vi "StandardEngineUI.vi"() -> ()   [LabVIEW 2013, in "Standard Engine Editor Node.lvclass"]
doc: "This VI is a template of the minimun components for a node UI.\nIt shows how to use the queue and the user event."
uses:
  Standard Engine Editor Node.lvclass
  <vilib>/NI/Configuration Framework/Node/NodeRef.ctl
  <vilib>/NI/Configuration Framework/Node/NISE_CEF_Node.lvclass
  <vilib>/NI/AMC/Message Queue.ctl
  <vilib>/NI/AMC/Message.ctl
  <vilib>/NI/Tools/Keyed Array/KeyedArray.ctl
  <vilib>/NI/Configuration Framework/Node/UserEventRef.ctl
  <vilib>/NI/Configuration Framework/Controls/EventCluster.ctl
  Execution Engine/Configuration/Supported Timing Sources.ctl
  Processor Assignment Mode.ctl
  Execution Engine/Configuration/Module Decimation.ctl
  Execution Engine/Configuration/timing reporting tags.ctl
  Execution Engine/Configuration/Error Actions By Category.ctl
  <vilib>/NI/Tag Bus Module Framework/runtime/error classification.ctl
  Execution Engine/Configuration/Error Actions.ctl
  <vilib>/NI/Tag Bus Data Framework/Configuration Editor/Classes/Engine Parent/Engine Parent Editor Node.lvclass
  Standard Engine Editor Node.lvclass/Standard Engine Editor Node.ctl
  Execution Engine/Configuration/Standard Engine Configuration.lvclass/Standard Engine Configuration.ctl
  Execution Engine/Configuration/Module Error Configuration.ctl
  Execution Engine/Configuration/Write Timing Source Type.vi
  Execution Engine/Configuration/Write Master Timing Module.vi
  Execution Engine/Configuration/Write Processor.vi
  Execution Engine/Configuration/Read Processor.vi
  Execution Engine/Configuration/Read Timing Source Type.vi
  <vilib>/NI/Tag Bus Data Framework/Configuration Editor/Classes/Engine Parent/Read Name.vi
  <vilib>/NI/AMC/Create Single Message.vi
  <vilib>/NI/AMC/Update Message Routing Info.vi
  <vilib>/NI/Configuration Framework/serializable configuration/get alias.vi
  Execution Engine/Configuration/Write Timing Source dt.vi
  Execution Engine/Configuration/Find Module Specific Config.vi
  <vilib>/Utility/error.llb/Error Cluster From Error Code.vi
  <vilib>/NI/Configuration Framework/error generator.vi
  <vilib>/NI/AMC/Send Message.vi
  Execution Engine/Configuration/Read Timing Source dt.vi
  <vilib>/NI/AMC/AMC.lvlib
  Execution Engine/Configuration/Standard Engine Configuration.lvclass
  <vilib>/NI/Tag Bus Module Framework/runtime/TBM module execution interface.lvclass
  <vilib>/NI/Configuration Framework/NISE_CEF_TreeControl.lvlib
  <vilib>/NI/Configuration Framework/serializable configuration/NISE_CEF_serializable configuration.lvclass
  <vilib>/NI/Tools/Keyed Array/Tools_KeyedArray.lvlib
panel:
  in  "Tab Control":T1(tab)
  in  "Enable Timing Report":bool
  in  "Module Timing Source":i32(listbox)
  in  "Engine Name":string
  in  "Timing Source dt":u32=5000
  in  "Timing Source Type":T2=enum."1 kHz Clock"
  in  "Procesor Assignment":i32 min=0
  in  "Mode":T3
  in  "Warning Message":string="This timing source is not deterministic."
  out "timing reporting":T4={"late index (bool)"="_stdeng_late", "late count index (U32)"="_stdeng_latecount", "current dt ns(U64)"="_stdeng_iteratedt"}
  in  "Report Errors?":bool
  out "error tag":string
  in  "Module to Configure":i32(listbox)
  in  "Module Decimation":T5={"Decimation"=1, "Offset"=0} {"Decimation" min=1}
  in  "Sort Order":i32
  in  "Async?":bool
  in  "Error Handling":T6[](array[typedef])
  in  "user event":T9
  in  "main queue":T10
  in  "node ref":T11
  # "Processor Assignment"
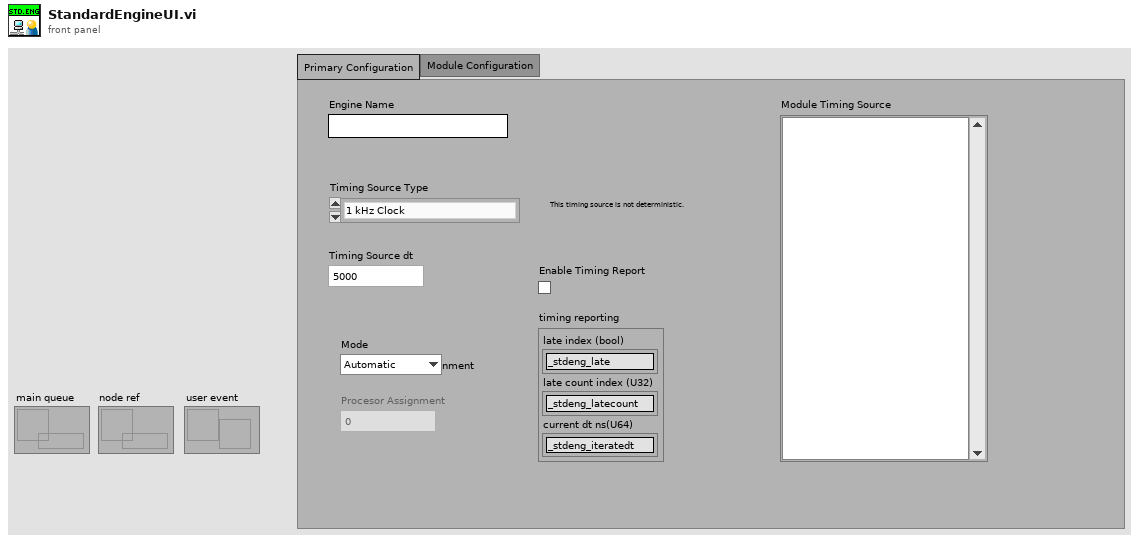
[diagram p1: front panel]
types:
  T1 = enum32{"Primary Configuration", "Module Configuration"}
  T2 = typedef "Standard Engine Configuration.lvclass/Supported Timing Sources.ctl" = enum16{"Use Module Timing Source", "1 kHz Clock", "1 MHz Clock", "Synchronize to Scan Engine"}
  T3 = typedef "Standard Engine Editor Node.lvclass/Processor Assignment Mode.ctl" = enum16{"Automatic", "Manual"}
  T4 = typedef "Standard Engine Configuration.lvclass/timing reporting tags.ctl" = cluster{"late index (bool)":string, "late count index (U32)":string, "current dt ns(U64)":string}
  T5 = typedef "Standard Engine Configuration.lvclass/Module Decimation.ctl" = cluster{"Decimation":u16, "Offset":u16}
  T6 = typedef "Standard Engine Configuration.lvclass/Error Actions By Category.ctl" = cluster{"error classification":T7, "Error Actions":T8[]}
  T7 = typedef "TBM module execution interface.lvclass/error classification.ctl" = enum16{"unknown", "none", "trivial", "recoverable", "critical"}
  T8 = typedef "Standard Engine Configuration.lvclass/Error Actions.ctl" = enum16{"Clear", "Notify", "Stop Component", "Stop Engine", "Safe State", "Attempt Recovery"}
  T9 = typedef "NISE_CEF_Node.lvclass/UserEventRef.ctl" = refnum<user-event>
  T10 = typedef "AMC.lvlib/Message Queue.ctl" = refnum<queue>
  T11 = typedef "NISE_CEF_Node.lvclass/NodeRef.ctl" = refnum<data-value>
  T12 = typedef "NISE_CEF_TreeControl.lvlib/EventCluster.ctl" = cluster{"command":string, "data":string}
  T13 = typedef "Standard Engine Configuration.lvclass/Module Error Configuration.ctl" = cluster{"Module Error Configuration":T6[]}
  T14 = enum8{"Enabled", "Disabled", "Disabled and Grayed Out"}
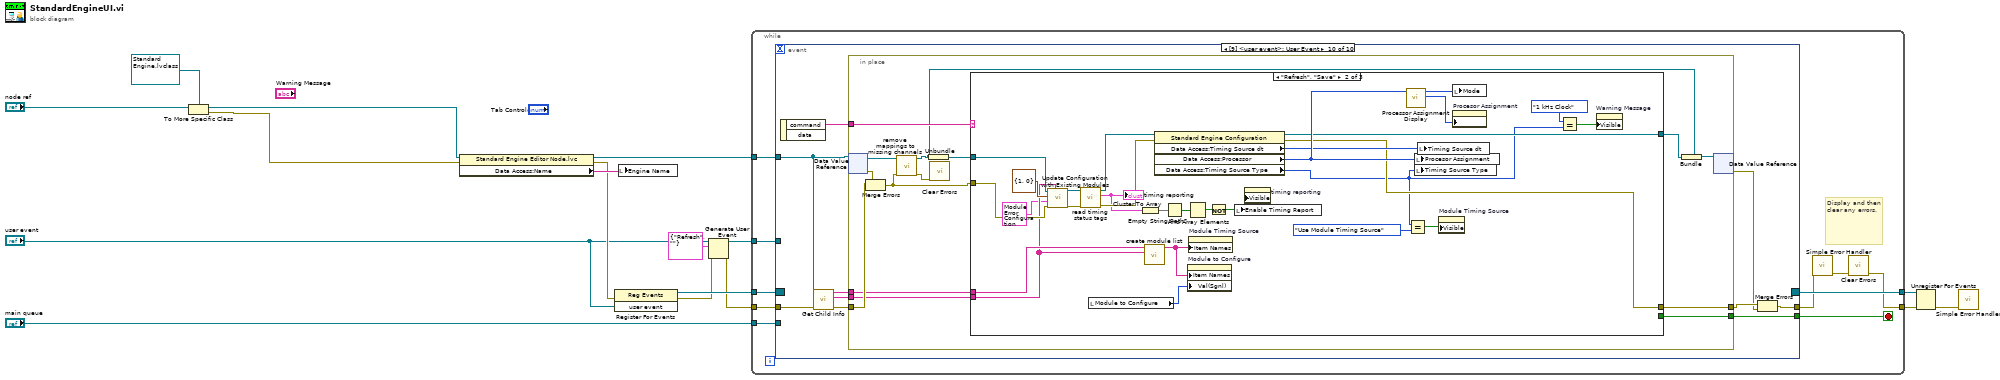
[diagram p0: block diagram]
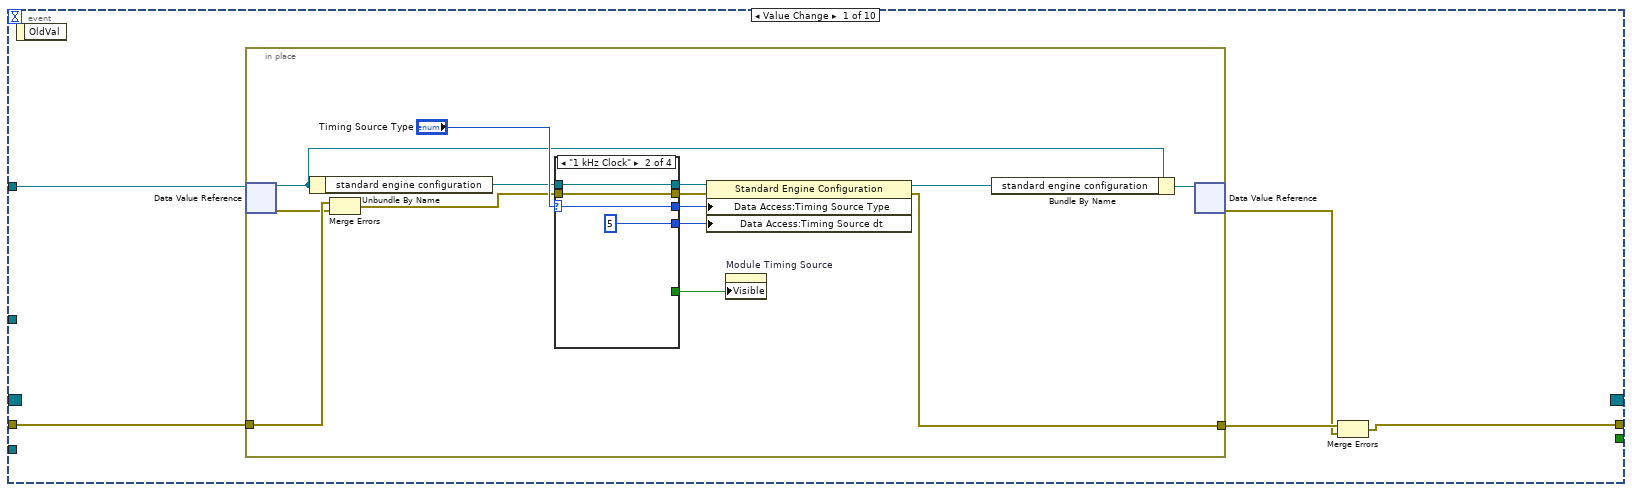
[diagram p2: hidden frame]
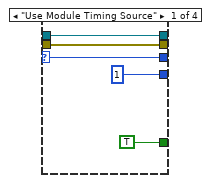
[diagram p3: hidden frame]
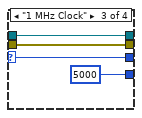
[diagram p4: hidden frame]
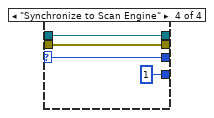
[diagram p5: hidden frame]
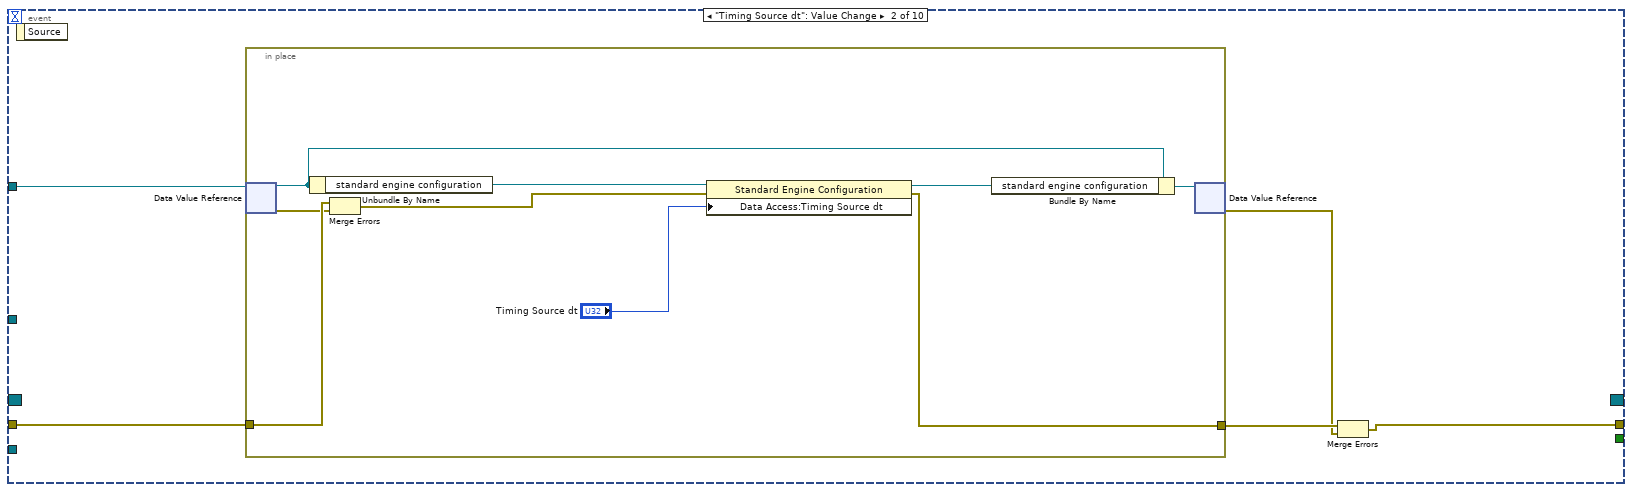
[diagram p6: hidden frame]
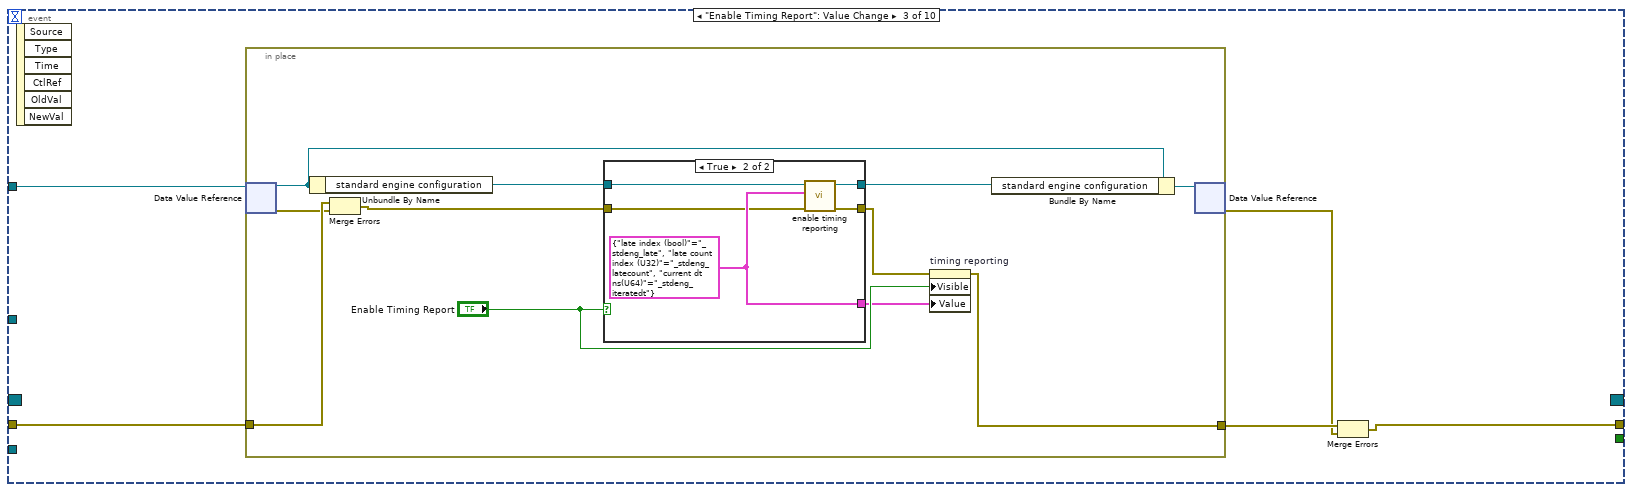
[diagram p7: hidden frame]
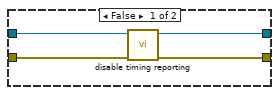
[diagram p8: hidden frame]
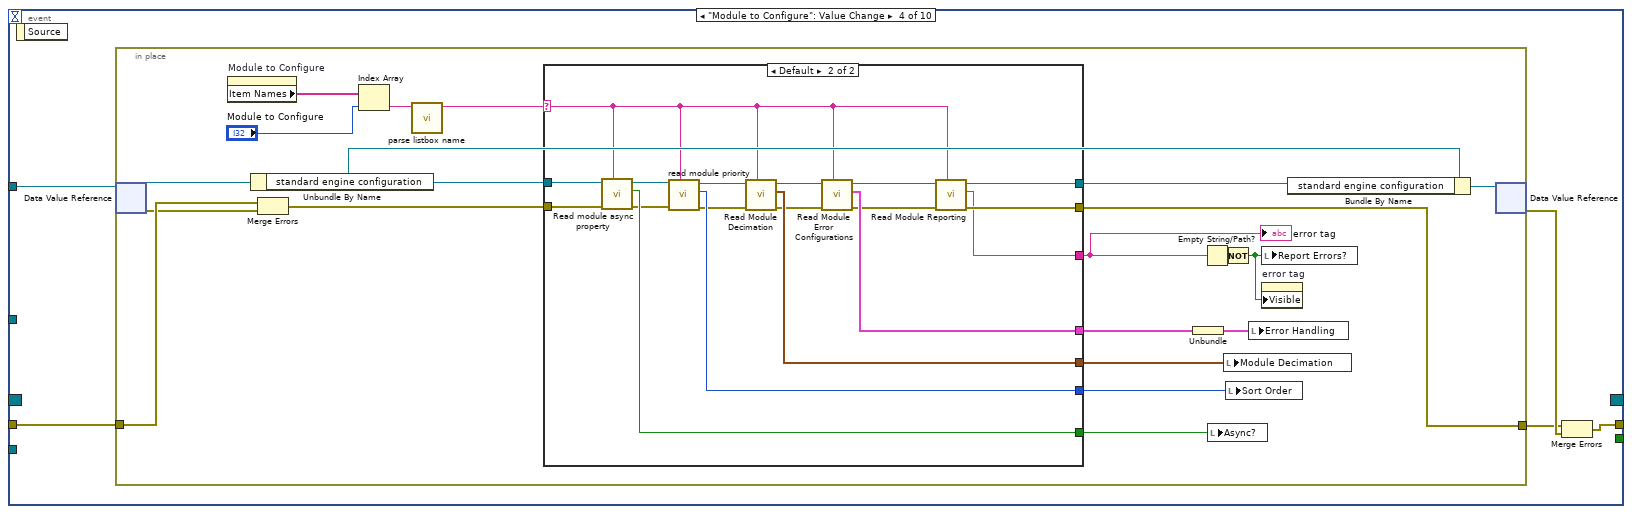
[diagram p9: hidden frame]
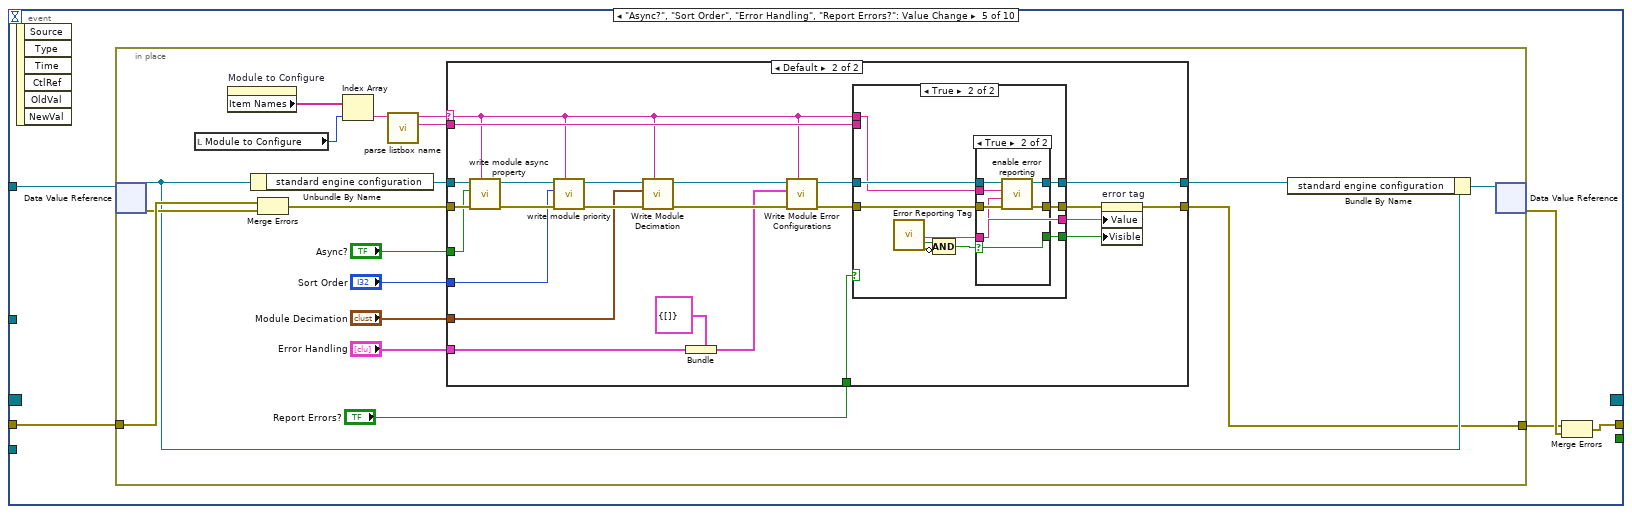
[diagram p11: hidden frame]
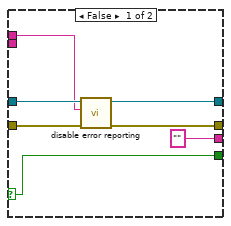
[diagram p13: hidden frame]
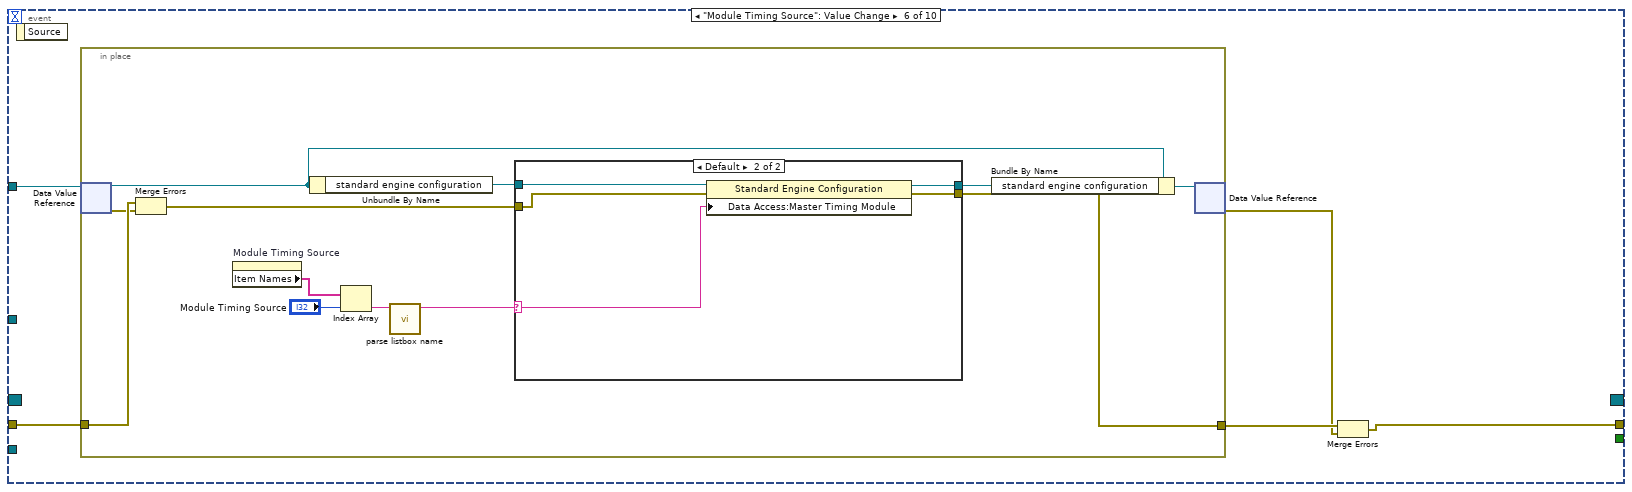
[diagram p15: hidden frame]
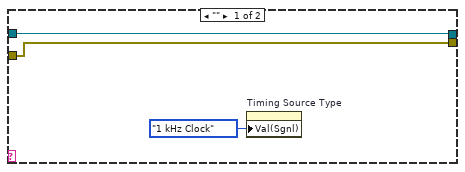
[diagram p16: hidden frame]
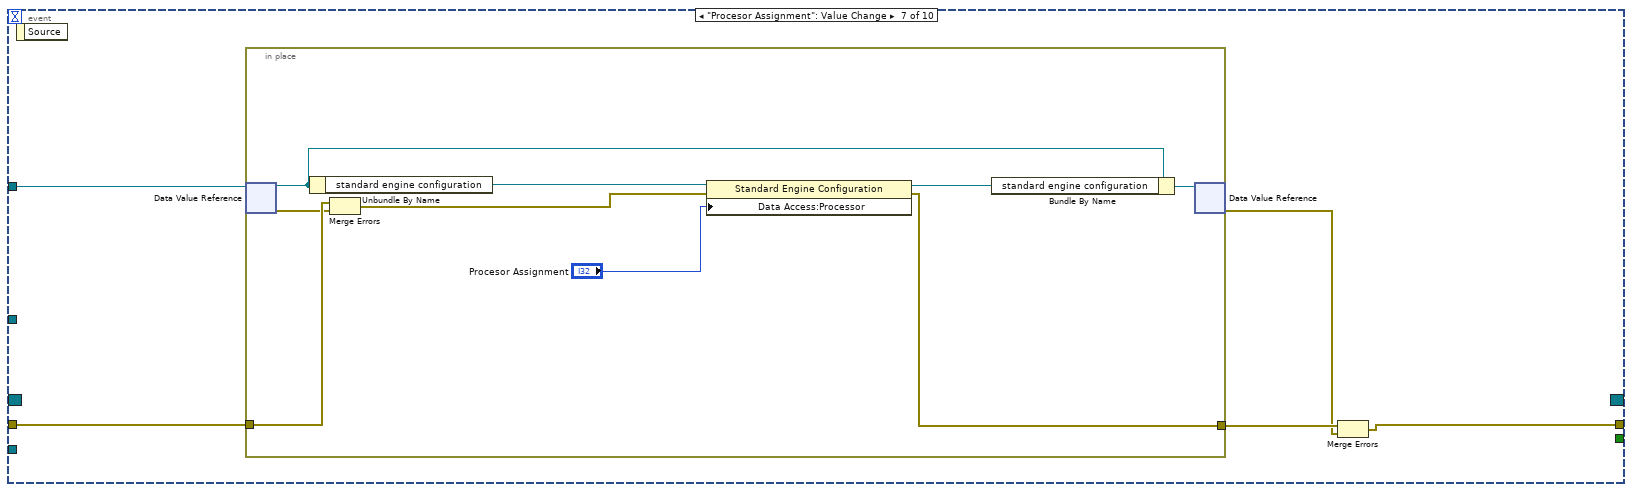
[diagram p17: hidden frame]
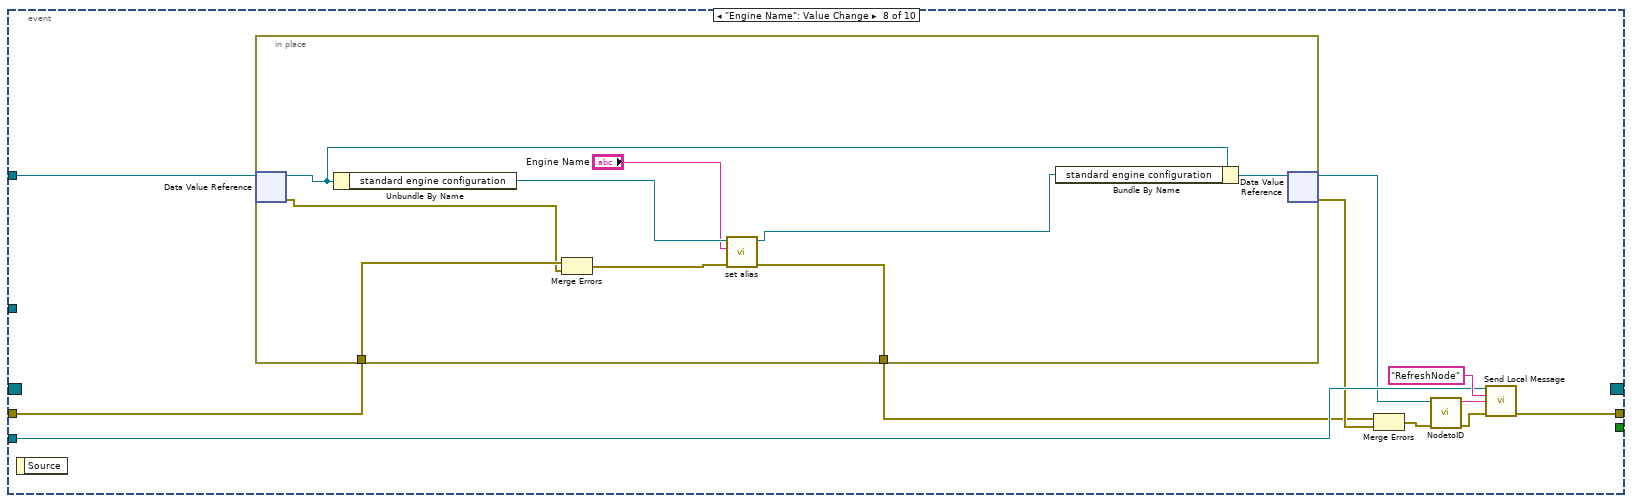
[diagram p18: hidden frame]
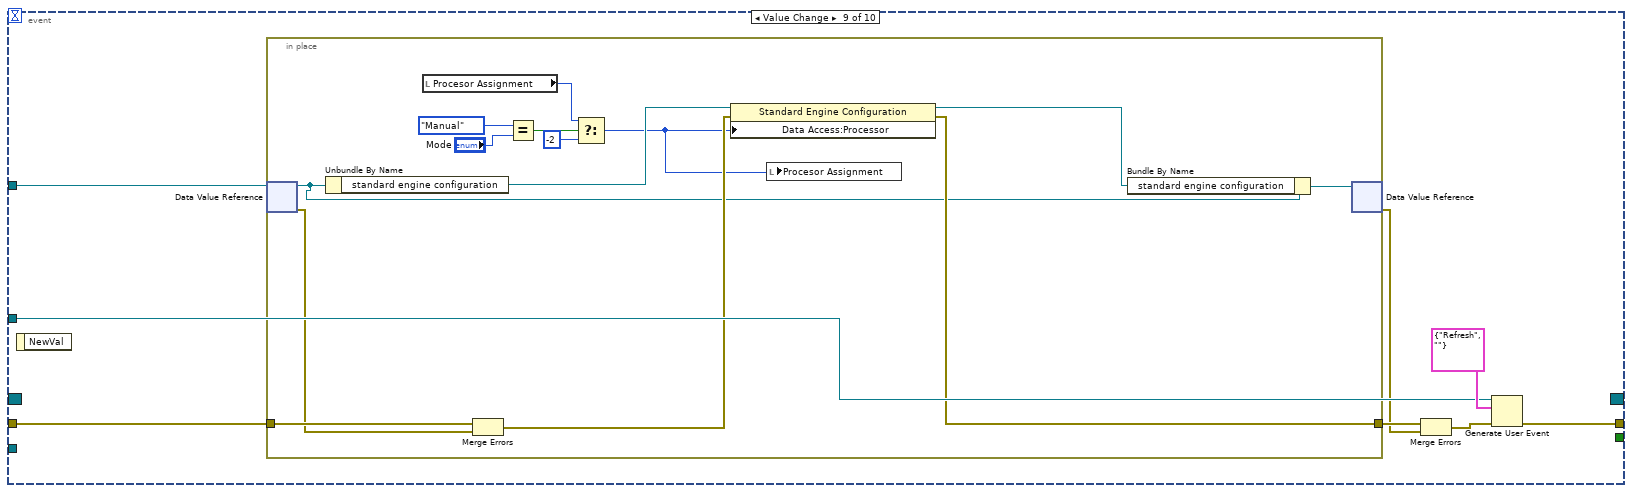
[diagram p19: hidden frame]
diagram:
  n1 = To More Specific Class(target class=refnum<data-value> refnum ("data value reference"), reference="node ref") -> (specific class reference=w12:refnum<data-value>, error out=w11:errorcluster)  [unwired: 1 in]
  n2 = property class="Standard Engine Editor Node.lvc"(reference=w12, error in=w11) -> (reference out=w8:refnum<data-value>, error out=w7:errorcluster, "Data Access:Name"=w13:string)
  n3 = register-events(error in=w7, "user event") -> (reference out=w16:refnum<event-registration>, error out=w6:errorcluster)  [unwired: 1 in]
  n4 = local write "Engine Name"(w13) -> ()
  n5 = Generate User Event(user event="user event", event data cluster=T12 {"command"="Refresh", "data"=""} ("event data"), error in=w6) -> (user event out=w3:T9, error out=w5:errorcluster)  [unwired: 1 in]
  n6 = while {
    tunnel: "main queue" -> [w27]
    tunnel: w16 -> [w26]
    tunnel: [w25] -> w15
    tunnel: [w19] -> w14
    tunnel: w5 -> [w23]
    tunnel: w8 -> [w22]
    tunnel: w3 -> [w18]
    stop <- w24 stop-if-true
    # "Display and then clear any errors."
    n7 = event shown="[9] <user event>: User Event" {
      selector: w26 -> [_ _ _ _ _ _ _ _ _ _]
      dyn-events: [_ _ _ _ _ _ _ _ _ _] -> w25
      timeout: _ -> [_ _ _ _ _ _ _ _ _ _]
      tunnel: w27 -> [_ _ _ _ _ _ _ w272 _ _]
      tunnel: [_ _ _ _ _ _ _ _ _ w314] -> w24
      tunnel: [w29 w65 w79 w105 w150 w225 w250 w270 w287 w306] -> w21
      tunnel: w23 -> [w32 w68 w82 w107 w152 w228 w253 w268 w286 w309]
      tunnel: w22 -> [w30 w66 w80 w106 w151 w226 w251 w267 w284 w307]
      tunnel: w18 -> [_ _ _ _ _ _ _ _ w289 _]
      event Value Change {
        n8 = event-data() -> ()  [unwired: 1 in, 1 out]
        n9 = in-place {
          in-place-border: w32 -> [w45]
          in-place-border: [w41] -> w31
          n10 = in-place-dvr #1(w30) -> (w36:refnum<class "Standard Engine Editor Node.lvclass">, w38:errorcluster)
          n11 = Unbundle By Name(w36) -> ("standard engine configuration"=w37:refnum<class "Standard Engine Configuration.lvclass">)
          n12 = Merge Errors(w45, w38) -> (w39:errorcluster)
          n13 = case shown="\"1 kHz Clock\"" "Timing Source Type" {
            selector: "Timing Source Type" -> [w51 w55 w57 w61]
            tunnel: w37 -> [w50 w54 w59 w63]
            tunnel: [w50 w54 w59 w63] -> w46
            tunnel: w39 -> [w49 w53 w58 w62]
            tunnel: [w49 w53 w58 w62] -> w44
            tunnel: [w51 w55 w57 w61] -> w40
            tunnel: [u32 1 ("Timing Source dt") u32 5 ("Timing Source dt") u32 5000 ("Timing Source dt") u32 1 ("Timing Source dt")] -> w42
            tunnel: [TRUE _ _ _] -> w33
            frame "Use Module Timing Source" {
            }
            frame "1 kHz Clock" {
            }
            frame "1 MHz Clock" {
            }
            frame "Synchronize to Scan Engine" {
            }
          }
          n14 = property class="Standard Engine Configuration"(reference=w46, error in=w44, "Data Access:Timing Source Type"=w40, "Data Access:Timing Source dt"=w42) -> (reference out=w34:refnum<class "Standard Engine Configuration.lvclass">, error out=w41:errorcluster)
          n15 = property on="Module Timing Source" class="LstBox (strict)"("Visible"=w33) -> ()  [unwired: 2 in, 2 out]
          n16 = Bundle By Name(cluster=w36, "standard engine configuration"=w34) -> (w35:refnum<class "Standard Engine Editor Node.lvclass">)
          n17 = in-place-dvr #1(w35) -> (w28:errorcluster)  [unwired: 1 out]
        }
        n18 = Merge Errors(w31, w28) -> (w29:errorcluster)
      }
      event "Timing Source dt": Value Change {
        n19 = event-data() -> ()  [unwired: 1 in, 1 out]
        n20 = in-place {
          in-place-border: w68 -> [w77]
          in-place-border: [w76] -> w67
          n21 = in-place-dvr #2(w66) -> (w72:refnum<class "Standard Engine Editor Node.lvclass">, w74:errorcluster)
          n22 = Unbundle By Name(w72) -> ("standard engine configuration"=w73:refnum<class "Standard Engine Configuration.lvclass">)
          n23 = Merge Errors(w77, w74) -> (w75:errorcluster)
          n24 = property class="Standard Engine Configuration"(reference=w73, error in=w75, "Data Access:Timing Source dt"="Timing Source dt") -> (reference out=w70:refnum<class "Standard Engine Configuration.lvclass">, error out=w76:errorcluster)
          n25 = Bundle By Name(cluster=w72, "standard engine configuration"=w70) -> (w71:refnum<class "Standard Engine Editor Node.lvclass">)
          n26 = in-place-dvr #2(w71) -> (w64:errorcluster)  [unwired: 1 out]
        }
        n27 = Merge Errors(w67, w64) -> (w65:errorcluster)
      }
      event "Enable Timing Report": Value Change {
        n28 = event-data() -> ()  [unwired: 1 in, 6 out]
        n29 = in-place {
          in-place-border: w82 -> [w93]
          in-place-border: [w89] -> w81
          n30 = in-place-dvr #3(w80) -> (w91:refnum<class "Standard Engine Editor Node.lvclass">, w92:errorcluster)
          n31 = Unbundle By Name(w91) -> ("standard engine configuration"=w87:refnum<class "Standard Engine Configuration.lvclass">)
          n32 = Merge Errors(w93, w92) -> (w84:errorcluster)
          n33 = case shown="True" "Enable Timing Report" {
            tunnel: w87 -> [w97 w102]
            tunnel: [w95 w101] -> w86
            tunnel: [_ w100] -> w85
            tunnel: w84 -> [w96 w99]
            tunnel: [w94 w98] -> w83
            frame False {
              n34 = call "disable timing reporting.vi"("error in"=w96, "Standard Engine Configuration in"=w97) -> ("error out"=w94:errorcluster, "Standard Engine Configuration out"=w95:refnum<class "Standard Engine Configuration.lvclass">)  [unwired: 8 in]
            }
            frame True {
              w100 = T4 {"late index (bool)"="_stdeng_late", "late count index (U32)"="_stdeng_latecount", "current dt ns(U64)"="_stdeng_iteratedt"} ("timing reporting")
              n35 = call "enable timing reporting.vi"("error in"=w99, "timing reporting"=w100, "Standard Engine Configuration in"=w102) -> ("error out"=w98:errorcluster, "Standard Engine Configuration out"=w101:refnum<class "Standard Engine Configuration.lvclass">)  [unwired: 7 in]
            }
          }
          n36 = property on="timing reporting" class="Clust (strict)"(error in=w83, "Visible"="Enable Timing Report", "Value"=w85) -> (error out=w89:errorcluster)  [unwired: 1 in, 1 out]
          n37 = Bundle By Name(cluster=w91, "standard engine configuration"=w86) -> (w90:refnum<class "Standard Engine Editor Node.lvclass">)
          n38 = in-place-dvr #3(w90) -> (w78:errorcluster)  [unwired: 1 out]
        }
        n39 = Merge Errors(w81, w78) -> (w79:errorcluster)
      }
      event "Module to Configure": Value Change {
        n40 = event-data() -> ()  [unwired: 1 in, 1 out]
        n41 = in-place {
          in-place-border: w107 -> [w127]
          in-place-border: [w112] -> w103
          n42 = in-place-dvr #4(w106) -> (w125:refnum<class "Standard Engine Editor Node.lvclass">, w126:errorcluster)
          n43 = property on="Module to Configure" class="LstBox (strict)"() -> ("Item Names"=w123:string[])  [unwired: 2 in, 2 out]
          n44 = Unbundle By Name(w125) -> ("standard engine configuration"=w120:refnum<class "Standard Engine Configuration.lvclass">)
          n45 = Merge Errors(w127, w126) -> (w119:errorcluster)
          n46 = Index Array(array=w123, index="Module to Configure") -> (element=w121:string)
          n47 = call "parse listbox name.vi"("formatted name"=w121) -> ("ID"=w108:string)  [unwired: 9 in, 1 out]
          n48 = case shown="Default" w108 {
            selector: w108 -> [_ w130]
            tunnel: w120 -> [w129 w147]
            tunnel: w119 -> [w128 w146]
            tunnel: [_ w145] -> w118
            tunnel: [_ w142] -> w117
            tunnel: [_ w139] -> w116
            tunnel: [_ w136] -> w115
            tunnel: [w128 w133] -> w112
            tunnel: [w129 w132] -> w111
            tunnel: [_ w131] -> w110
            frame "" {
            }
            frame Default {
              n49 = call "Read module async property.vi"("Module ID"=w130, "error in"=w146, "Standard Engine Repo Data in"=w147) -> ("error out"=w143:errorcluster, "async?"=w145:bool, "Standard Engine Repo Data out"=w144:refnum<class "Standard Engine Configuration.lvclass">)  [unwired: 6 in]
              n50 = call "read module priority.vi"("Module ID"=w130, "error in"=w143, "Standard Engine Repo Data in"=w144) -> ("error out"=w141:errorcluster, "execution order priority"=w142:i32, "Standard Engine Repo Data out"=w140:refnum<class "Standard Engine Configuration.lvclass">)  [unwired: 6 in]
              n51 = call "Read Module Decimation.vi"("Module ID"=w130, "error in"=w141, "Standard Engine Repo Data in"=w140) -> ("error out"=w137:errorcluster, "Module Decimation"=w139:T5, "Standard Engine Repo Data out"=w138:refnum<class "Standard Engine Configuration.lvclass">)  [unwired: 6 in]
              n52 = call "Read Module Error Configurations.vi"("Module ID"=w130, "error in"=w137, "Standard Engine Repo Data in"=w138) -> ("error out"=w134:errorcluster, "Module Error Configuration"=w136:T13, "Standard Engine Repo Data out"=w135:refnum<class "Standard Engine Configuration.lvclass">)  [unwired: 6 in]
              n53 = call "Read Module Reporting.vi"("Module ID"=w130, "error in"=w134, "Standard Engine Repo Data in"=w135) -> ("error out"=w133:errorcluster, "error tag"=w131:string, "Standard Engine Repo Data out"=w132:refnum<class "Standard Engine Configuration.lvclass">)  [unwired: 6 in]
            }
          }
          "error tag" <- w110
          n54 = Unbundle(w115) -> ("Module Error Configuration"=w114:T6[])
          n55 = Empty String/Path?(string/path=w110) -> (empty?=w113:bool)
          n56 = local write "Async?"(w118) -> ()
          n57 = Not(x=w113) -> (.not. x?=w109:bool)
          n58 = local write "Module Decimation"(w116) -> ()
          n59 = local write "Sort Order"(w117) -> ()
          n60 = local write "Error Handling"(w114) -> ()
          n61 = local write "Report Errors?"(w109) -> ()
          n62 = property on="error tag" class="Str"("Visible"=w109) -> ()  [unwired: 2 in, 2 out]
          n63 = Bundle By Name(cluster=w125, "standard engine configuration"=w111) -> (w124:refnum<class "Standard Engine Editor Node.lvclass">)
          n64 = in-place-dvr #4(w124) -> (w104:errorcluster)  [unwired: 1 out]
        }
        n65 = Merge Errors(w103, w104) -> (w105:errorcluster)
      }
      event "Async?", "Sort Order", "Error Handling", "Report Errors?": Value Change {
        n66 = event-data() -> ()  [unwired: 1 in, 6 out]
        n67 = in-place {
          in-place-border: w152 -> [w170]
          in-place-border: [w156] -> w148
          n68 = in-place-dvr #5(w151) -> (w168:refnum<class "Standard Engine Editor Node.lvclass">, w169:errorcluster)
          n69 = local read "Module to Configure"() -> (w159:i32)
          n70 = property on="Module to Configure" class="LstBox (strict)"() -> ("Item Names"=w166:string[])  [unwired: 2 in, 2 out]
          n71 = Unbundle By Name(w168) -> ("standard engine configuration"=w164:refnum<class "Standard Engine Configuration.lvclass">)
          n72 = Merge Errors(w170, w169) -> (w163:errorcluster)
          n73 = Index Array(array=w166, index=w159) -> (element=w165:string)
          n74 = call "parse listbox name.vi"("formatted name"=w165) -> ("display"=w154:string, "ID"=w153:string)  [unwired: 9 in]
          n75 = case shown="Default" w153 {
            selector: w153 -> [_ w174]
            tunnel: w164 -> [w172 w196]
            tunnel: w163 -> [w171 w195]
            tunnel: "Async?" -> [_ w190]
            tunnel: "Sort Order" -> [_ w189]
            tunnel: "Module Decimation" -> [_ w188]
            tunnel: [w172 w183] -> w158
            tunnel: "Error Handling" -> [_ w181]
            tunnel: [w171 w179] -> w156
            tunnel: "Report Errors?" -> [_ w177]
            tunnel: w154 -> [_ w175]
            frame "" {
            }
            frame Default {
              n76 = call "write module async property.vi"("Module ID"=w174, "error in"=w195, "async?"=w190, "Standard Engine Repo Data in"=w196) -> ("error out"=w193:errorcluster, "Standard Engine Repo Data out"=w194:refnum<class "Standard Engine Configuration.lvclass">)  [unwired: 6 in]
              n77 = call "write module priority.vi"("Module ID"=w174, "error in"=w193, "execution order priority"=w189, "Standard Engine Repo Data in"=w194) -> ("error out"=w191:errorcluster, "Standard Engine Repo Data out"=w192:refnum<class "Standard Engine Configuration.lvclass">)  [unwired: 6 in]
              n78 = call "Write Module Decimation.vi"("Module ID"=w174, "error in"=w191, "Module Decimation"=w188, "Standard Engine Repo Data in"=w192) -> ("error out"=w186:errorcluster, "Standard Engine Repo Data out"=w187:refnum<class "Standard Engine Configuration.lvclass">)  [unwired: 6 in]
              n79 = Bundle(cluster=T13 {"Module Error Configuration"=[]} ("Module Error Configuration"), "Module Error Configuration"=w181) -> (w180:T13)
              n80 = call "Write Module Error Configurations.vi"("Module ID"=w174, "error in"=w186, "Module Error Configuration"=w180, "Standard Engine Repo Data in"=w187) -> ("error out"=w184:errorcluster, "Standard Engine Repo Data out"=w185:refnum<class "Standard Engine Configuration.lvclass">)  [unwired: 6 in]
              n81 = case shown="True" w177 {
                selector: w177 -> [w197 _]
                tunnel: w185 -> [w203 w213]
                tunnel: w184 -> [w202 w212]
                tunnel: [w200 w211] -> w183
                tunnel: [w201 w210] -> w178
                tunnel: w174 -> [w199 w209]
                tunnel: ["" w208] -> w176
                tunnel: w175 -> [_ _]
                tunnel: [w197 w204] -> w173
                frame False {
                  n82 = call "disable error reporting.vi"("error in"=w202, "module ID"=w199, "Standard Engine Configuration in"=w203) -> ("error out"=w201:errorcluster, "Standard Engine Configuration out"=w200:refnum<class "Standard Engine Configuration.lvclass">)  [unwired: 7 in]
                }
                frame True {
                  n83 = call "Error Reporting Tag"() -> ("Tag Name"=w208:string, "OK"=w207:bool, "error out"=w206:errorcluster)  [unwired: 17 in]
                  n84 = Compound Arithmetic op=AND(w207, invert w206) -> (w205:bool)
                  n85 = case shown="True" w205 {
                    selector: w205 -> [w214 w217]
                    tunnel: w213 -> [w216 w223]
                    tunnel: w212 -> [w215 w222]
                    tunnel: [w216 w221] -> w211
                    tunnel: [w215 w220] -> w210
                    tunnel: w209 -> [_ w219]
                    tunnel: w208 -> [_ w218]
                    tunnel: [w214 w217] -> w204
                    frame False {
                    }
                    frame True {
                      n86 = call "enable error reporting.vi"("error in"=w222, "tag"=w218, "module ID"=w219, "Standard Engine Configuration in"=w223) -> ("error out"=w220:errorcluster, "Standard Engine Configuration out"=w221:refnum<class "Standard Engine Configuration.lvclass">)  [unwired: 6 in]
                    }
                  }
                }
              }
              n87 = property on="error tag" class="Str"(error in=w178, "Value"=w176, "Visible"=w173) -> (error out=w179:errorcluster)  [unwired: 1 in, 1 out]
            }
          }
          n88 = Bundle By Name(cluster=w168, "standard engine configuration"=w158) -> (w167:refnum<class "Standard Engine Editor Node.lvclass">)
          n89 = in-place-dvr #5(w167) -> (w149:errorcluster)  [unwired: 1 out]
        }
        n90 = Merge Errors(w148, w149) -> (w150:errorcluster)
      }
      event "Module Timing Source": Value Change {
        n91 = event-data() -> ()  [unwired: 1 in, 1 out]
        n92 = in-place {
          in-place-border: w228 -> [w240]
          in-place-border: [w239] -> w227
          n93 = in-place-dvr #6(w226) -> (w235:refnum<class "Standard Engine Editor Node.lvclass">, w237:errorcluster)
          n94 = Merge Errors(w240, w237) -> (w238:errorcluster)
          n95 = property on="Module Timing Source" class="LstBox (strict)"() -> ("Item Names"=w231:string[])  [unwired: 2 in, 2 out]
          n96 = Unbundle By Name(w235) -> ("standard engine configuration"=w236:refnum<class "Standard Engine Configuration.lvclass">)
          n97 = Index Array(array=w231, index="Module Timing Source") -> (element=w230:string)
          n98 = call "parse listbox name.vi"("formatted name"=w230) -> ("ID"=w229:string)  [unwired: 9 in, 1 out]
          n99 = case shown="Default" w229 {
            selector: w229 -> [_ w244]
            tunnel: [w243 w248] -> w239
            tunnel: w238 -> [w243 w247]
            tunnel: w236 -> [w242 w246]
            tunnel: [w242 w245] -> w233
            frame "" {
              n100 = property on="Timing Source Type" class="Enum (strict)"("Val(Sgnl)"=Supported_Timing_Sources."1 kHz Clock" ("Value (Signaling)")) -> ()  [unwired: 2 in, 2 out]
            }
            frame Default {
              n101 = property class="Standard Engine Configuration"(reference=w246, error in=w247, "Data Access:Master Timing Module"=w244) -> (reference out=w245:refnum<class "Standard Engine Configuration.lvclass">, error out=w248:errorcluster)
            }
          }
          n102 = Bundle By Name(cluster=w235, "standard engine configuration"=w233) -> (w234:refnum<class "Standard Engine Editor Node.lvclass">)
          n103 = in-place-dvr #6(w234) -> (w224:errorcluster)  [unwired: 1 out]
        }
        n104 = Merge Errors(w227, w224) -> (w225:errorcluster)
      }
      event "Procesor Assignment": Value Change {
        n105 = event-data() -> ()  [unwired: 1 in, 1 out]
        n106 = in-place {
          in-place-border: w253 -> [w262]
          in-place-border: [w261] -> w252
          n107 = in-place-dvr #7(w251) -> (w257:refnum<class "Standard Engine Editor Node.lvclass">, w259:errorcluster)
          n108 = Unbundle By Name(w257) -> ("standard engine configuration"=w258:refnum<class "Standard Engine Configuration.lvclass">)
          n109 = Merge Errors(w262, w259) -> (w260:errorcluster)
          n110 = property class="Standard Engine Configuration"(reference=w258, error in=w260, "Data Access:Processor"="Procesor Assignment") -> (reference out=w255:refnum<class "Standard Engine Configuration.lvclass">, error out=w261:errorcluster)
          n111 = Bundle By Name(cluster=w257, "standard engine configuration"=w255) -> (w256:refnum<class "Standard Engine Editor Node.lvclass">)
          n112 = in-place-dvr #7(w256) -> (w249:errorcluster)  [unwired: 1 out]
        }
        n113 = Merge Errors(w252, w249) -> (w250:errorcluster)
      }
      event "Engine Name": Value Change {
        n114 = event-data() -> ()  [unwired: 1 in, 1 out]
        n115 = in-place {
          in-place-border: w268 -> [w282]
          in-place-border: [w277] -> w263
          n116 = in-place-dvr #8(w267) -> (w281:refnum<class "Standard Engine Editor Node.lvclass">, w279:errorcluster)
          n117 = Unbundle By Name(w281) -> ("standard engine configuration"=w275:refnum<class "Standard Engine Configuration.lvclass">)
          n118 = Merge Errors(w282, w279) -> (w278:errorcluster)
          n119 = call <vilib>:"set alias.vi"("error in"=w278, "alias"="Engine Name", "configuration in"=w275) -> ("error out"=w277:errorcluster, "configuration out"=w276:refnum<class "Standard Engine Configuration.lvclass">)  [unwired: 7 in]
          n120 = Bundle By Name(cluster=w281, "standard engine configuration"=w276) -> (w280:refnum<class "Standard Engine Editor Node.lvclass">)
          n121 = in-place-dvr #8(w280) -> (w266:refnum<data-value>, w265:errorcluster)
        }
        n122 = Merge Errors(w263, w265) -> (w264:errorcluster)
        n123 = call <vilib>:"NodetoID.vi"("error in"=w264, "node ref"=w266) -> ("error out"=w269:errorcluster, "ID"=w271:string)  [unwired: 8 in]
        n124 = call <vilib>:"Send Local Message.vi"("message queue in"=w272, "message name"="RefreshNode" ("Message Name"), "message value"=w271, "error in"=w269) -> ("error out"=w270:errorcluster)  [unwired: 9 in, 2 out]
      }
      event Value Change {
        n125 = event-data() -> ()  [unwired: 1 in, 1 out]
        n126 = in-place {
          in-place-border: [w300] -> w288
          in-place-border: w286 -> [w299]
          n127 = in-place-dvr #9(w284) -> (w296:refnum<class "Standard Engine Editor Node.lvclass">, w297:errorcluster)
          n128 = Unbundle By Name(w296) -> ("standard engine configuration"=w293:refnum<class "Standard Engine Configuration.lvclass">)
          n129 = local read "Procesor Assignment"() -> (w292:i32)
          n130 = Merge Errors(w299, w297) -> (w298:errorcluster)
          n131 = Equal?(x=Processor_Assignment_Mode."Manual", y="Mode") -> (x = y?=w301:bool)
          n132 = Select(t=w292, s=w301, f=-2 ("Processor")) -> (s? t:f=w291:i32)
          n133 = property class="Standard Engine Configuration"(reference=w293, error in=w298, "Data Access:Processor"=w291) -> (reference out=w294:refnum<class "Standard Engine Configuration.lvclass">, error out=w300:errorcluster)
          n134 = local write "Procesor Assignment"(w291) -> ()
          n135 = Bundle By Name(cluster=w296, "standard engine configuration"=w294) -> (w295:refnum<class "Standard Engine Editor Node.lvclass">)
          n136 = in-place-dvr #9(w295) -> (w283:errorcluster)  [unwired: 1 out]
        }
        n137 = Merge Errors(w288, w283) -> (w285:errorcluster)
        n138 = Generate User Event(user event=w289, event data cluster=T12 {"command"="Refresh", "data"=""} ("event data"), error in=w285) -> (error out=w287:errorcluster)  [unwired: 1 in, 1 out]
      }
      event User Event {
        n139 = event-data() -> ("command"=w312:string)  [unwired: 1 in, 1 out]
        n140 = call "Get Child Info.vi"("error in (no error)"=w309, "Data Value Reference in"=w307) -> ("error out"=w308:errorcluster, "Instance Identifier"=w310:string[], "Display Names"=w311:string[])  [unwired: 7 in]
        n141 = in-place {
          in-place-border: [w328] -> w314
          in-place-border: w308 -> [w327]
          in-place-border: [w326] -> w313
          in-place-border: w312 -> [w325]
          in-place-border: w311 -> [w324]
          in-place-border: w310 -> [w323]
          n142 = in-place-dvr #10(w307) -> (w317:refnum<class "Standard Engine Editor Node.lvclass">, w322:errorcluster)
          n143 = Merge Errors(w327, w322) -> (w316:errorcluster)
          n144 = call <vilib>:"remove mappings to missing channels.vi"("error in"=w316, "Engine Parent Editor Node in"=w317) -> ("error out"=w315:errorcluster, "Engine Parent Editor Node out"=w318:refnum<class "Standard Engine Editor Node.lvclass">)  [unwired: 8 in]
          n145 = Unbundle(w318) -> (w321:refnum<class "Standard Engine Configuration.lvclass">)
          n146 = call <vilib>:"Clear Errors.vi"("error in (no error)"=w315) -> ()  [unwired: 6 in, 1 out]
          n147 = case shown="\"Refresh\", \"Save\"" w325 {
            tunnel: [_ _ TRUE] -> w328
            tunnel: w316 -> [w330 w349 w360]
            tunnel: [w330 w351 w360] -> w326
            tunnel: w321 -> [w329 w350 w359]
            tunnel: w324 -> [_ w347 _]
            tunnel: w323 -> [_ w346 _]
            tunnel: [w329 w348 w359] -> w319
            frame Default {
            }
            frame "Refresh", "Save" {
              n148 = call "Update Configuration with Existing Modules.vi"("Module IDs"=w346, "error in"=w349, "Default Module Error Configuration"=T13 {"Module Error Configuration"=[{"error classification"=enum."unknown", "Error Actions"=[enum."Stop Component"]}, {"error classification"=enum."none", "Error Actions"=[enum."Clear"]}, {"error classification"=enum."trivial", "Error Actions"=[enum."Notify"]}, {"error classification"=enum."recoverable", "Error Actions"=[enum."Attempt Recovery"]}, {"error classification"=enum."critical", "Error Actions"=[enum."Stop Engine"]}]} ("Module Error Configuration"), "Default Module Decimation"=T5 {"Decimation"=1, "Offset"=0}, "Standard Engine Configuration in"=w350) -> ("error out"=w343:errorcluster, "Standard Engine Configuration out"=w342:refnum<class "Standard Engine Configuration.lvclass">)  [unwired: 5 in]
              n149 = call "read timing status tags.vi"("error in"=w343, "Standard Engine Configuration in"=w342) -> ("error out"=w340:errorcluster, "timing reporting"=w339:T4, "Standard Engine Configuration out"=w341:refnum<class "Standard Engine Configuration.lvclass">)  [unwired: 7 in]
              "timing reporting" <- w339
              n150 = local read "Module to Configure"() -> (w344:i32)
              n151 = Cluster To Array(cluster=w339) -> (array=w338:string[])
              n152 = call "create module list.vi"("Instance Identifier"=w346, "Display Names"=w347) -> ("listbox names"=w345:string[])  [unwired: 9 in]
              n153 = property class="Standard Engine Configuration"(reference=w341, error in=w340) -> (reference out=w348:refnum<class "Standard Engine Configuration.lvclass">, error out=w351:errorcluster, "Data Access:Timing Source dt"=w352:u32, "Data Access:Processor"=w353:i32, "Data Access:Timing Source Type"=w333:T2)
              n154 = Empty String/Path?(string/path=w338) -> (empty?=w337:bool[])
              n155 = And Array Elements(Boolean array=w337) -> (logical AND=w336:bool)
              n156 = property on="Module to Configure" class="LstBox (strict)"("Item Names"=w345, "Val(Sgnl)"=w344) -> ()  [unwired: 2 in, 2 out]
              n157 = property on="Module Timing Source" class="LstBox (strict)"("Item Names"=w345) -> ()  [unwired: 2 in, 2 out]
              n158 = Not(x=w336) -> (.not. x?=w335:bool)
              n159 = local write "Enable Timing Report"(w335) -> ()
              n160 = property on="timing reporting" class="Clust (strict)"("Visible"=w335) -> ()  [unwired: 2 in, 2 out]
              n161 = call "Processor Assignment Display.vi"("Data Access:Processor"=w353) -> ("Enabled?"=w355:T14, "Mode"=w354:T3)  [unwired: 9 in]
              n162 = Equal?(x=w333, y=Supported_Timing_Sources."Use Module Timing Source") -> (x = y?=w331:bool)
              n163 = local write "Procesor Assignment"(w353) -> ()
              n164 = local write "Timing Source Type"(w333) -> ()
              n165 = local write "Timing Source dt"(w352) -> ()
              n166 = property on="Module Timing Source" class="LstBox (strict)"("Visible"=w331) -> ()  [unwired: 2 in, 2 out]
              n167 = local write "Mode"(w354) -> ()
              n168 = property on="Procesor Assignment" class="DigNum (strict)"("DisabledEnum"=w355) -> ()  [unwired: 2 in, 2 out]
              n169 = Equal?(x=Supported_Timing_Sources."1 kHz Clock" ("Timing Source Type"), y=w333) -> (x = y?=w356:bool)
              n170 = property on="Warning Message" class="Str"("Visible"=w356) -> ()  [unwired: 2 in, 2 out]
            }
            frame "Stop" {
            }
          }
          n171 = Bundle(cluster=w318, w319) -> (w320:refnum<class "Standard Engine Editor Node.lvclass">)
          n172 = in-place-dvr #10(w320) -> (w305:errorcluster)  [unwired: 1 out]
        }
        n173 = Merge Errors(w313, w305) -> (w306:errorcluster)
      }
    }
    n174 = call <vilib>:"Simple Error Handler.vi"("error in (no error)"=w21) -> ("error out"=w20:errorcluster)  [unwired: 4 in, 4 out]
    n175 = call <vilib>:"Clear Errors.vi"("error in (no error)"=w20) -> ("error out"=w19:errorcluster)  [unwired: 6 in]
  }
  n176 = Unregister For Events(event registration refnum=w15, error in=w14) -> (error out=w10:errorcluster)
  n177 = call <vilib>:"Simple Error Handler.vi"("error in (no error)"=w10) -> ()  [unwired: 4 in, 5 out]
